vi "ConvertStatusFromNumericToString.vi"(11 "Protect Status":i32) -> (3 "Numeric Indicator":string)   [LabVIEW 2018, in "AcPwrPlugins.lvlib" / "ChromaAcLoad.lvclass"]
uses:
  ChromaAcLoad.lvclass
panel:
  in  "String 2":string="This command returns the status of electronic load.\n\nGetting Parameter:\n\n1:Under frequency range or over frequency range.\n\n2|4:AC Mode voltage is lower than 45V, DC Mode voltage is lower than 7.5V.\n\n8:AC Mode voltage is higher than 350V.\n\n16:Voltage overshooting, Vpeak is higher than 600V.\n\n32:AC/DC Mode current is higher than 18A(63803) or 45A(63804).\n\n64:AC/DC Mode power is higher than 1800W(63803)or 4500W (63804).\n\n128:Over temperature protection.\n\n256:Fan fail.\n\n512:Load fail.\n\n1024:Under frequency range or over frequency range.\n"
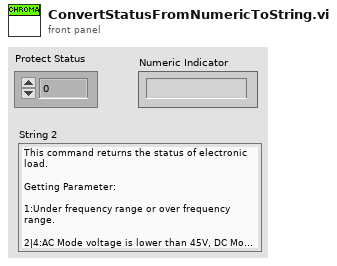
[diagram p1: front panel]
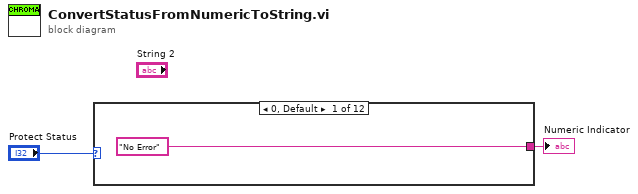
[diagram p0: block diagram]
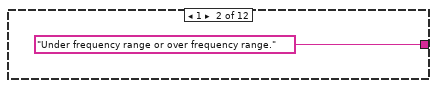
[diagram p2: hidden frame]
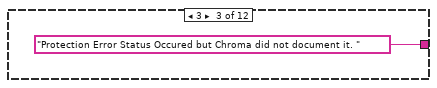
[diagram p3: hidden frame]
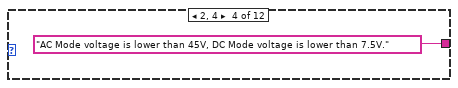
[diagram p4: hidden frame]
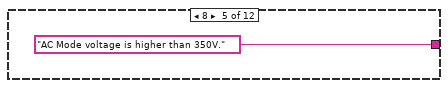
[diagram p5: hidden frame]
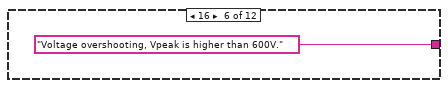
[diagram p6: hidden frame]
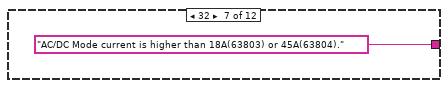
[diagram p7: hidden frame]
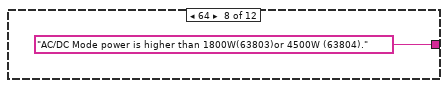
[diagram p8: hidden frame]
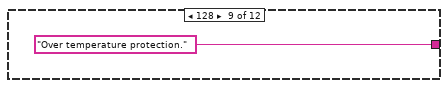
[diagram p9: hidden frame]
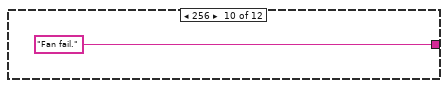
[diagram p10: hidden frame]
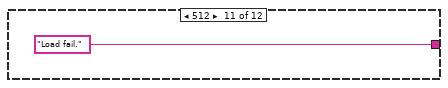
[diagram p11: hidden frame]
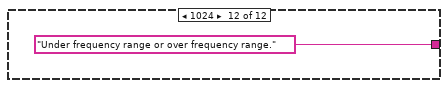
[diagram p12: hidden frame]
diagram:
  n1 = case shown="0, Default" "Protect Status" {
    tunnel: ["No Error" "Under frequency range or over frequency range." "Protection Error Status Occured but Chroma did not document it. " "AC Mode voltage is lower than 45V, DC Mode voltage is lower than 7.5V." "AC Mode voltage is higher than 350V." "Voltage overshooting, Vpeak is higher than 600V." "AC/DC Mode current is higher than 18A(63803) or 45A(63804)." "AC/DC Mode power is higher than 1800W(63803)or 4500W (63804)." "Over temperature protection." "Fan fail." "Load fail." "Under frequency range or over frequency range."] -> w1
    frame 0, Default {
    }
    frame 1 {
    }
    frame 3 {
    }
    frame 2, 4 {
    }
    frame 8 {
    }
    frame 16 {
    }
    frame 32 {
    }
    frame 64 {
    }
    frame 128 {
    }
    frame 256 {
    }
    frame 512 {
    }
    frame 1024 {
    }
  }
  "Numeric Indicator" <- w1
